vi "Connect Core.vi"(4 "queueRef":refnum<queue>, 5 "Commit Only?":bool, 6 "Access (R/W allowed)":T1, 7 "Mode (buffer)":u16(ring)=1 items=["commit", "buffer"], 8 "Error In":errorcluster, 11 "SVConnection in":refnum<class "DSConnection.lvclass">) -> (0 "Error Out":errorcluster, 3 "SVConnection out":refnum<class "DSConnection.lvclass">)   [LabVIEW 2015, in "CS++ProcessVariables.lvlib" / "DSConnection.lvclass"]
doc: "Open reference to a data socket item if not already connected."
uses:
  DSConnection.lvclass
  DSConnection.lvclass/DSConnection.ctl
  PVConnection/PVConnection.lvclass/PVConnection.ctl
  ProcessVariable/PV.lvclass/PV.ctl
  ProcessVariable/PV.lvclass
  PVConnection/PVConnection.lvclass
  Libraries/Utilities/CS++Utilities.lvlib
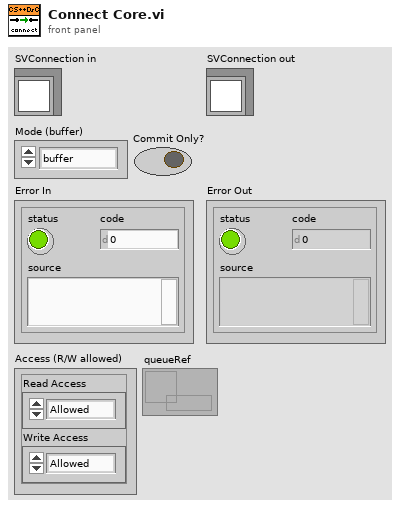
[diagram p1: front panel]
types:
  T1 = cluster{"Read Access":enum8{"Allowed", "Required", "None"}, "Write Access":enum8{"Allowed", "Required", "None"}}
  T2 = enum16{"Read", "Write", "ReadWrite", "BufferedRead", "BufferedReadWrite"}
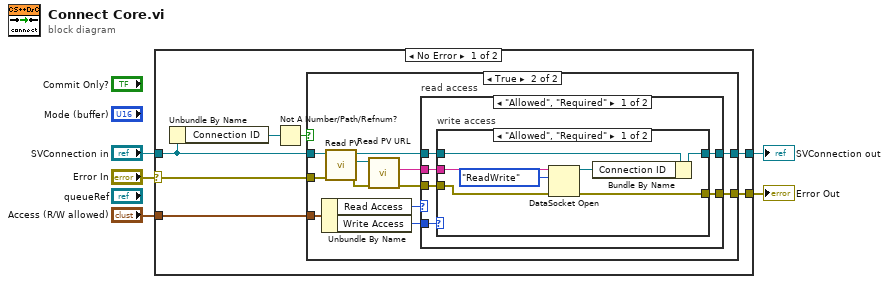
[diagram p0: block diagram]
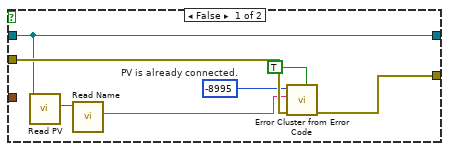
[diagram p2: hidden frame]
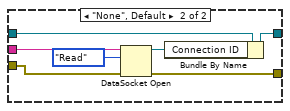
[diagram p3: hidden frame]
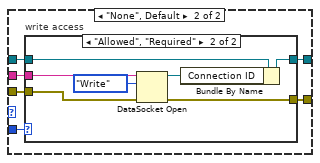
[diagram p4: hidden frame]
diagram:
  n1 = case shown="No Error" "Error In" {
    selector: "Error In" -> [w12 w68]
    tunnel: [w11 w68] -> w4
    tunnel: [w10 w67] -> w2
    tunnel: "SVConnection in" -> [w7 w67]
    tunnel: "Access (R/W allowed)" -> [w8 _]
    frame No Error {
      n2 = Unbundle By Name(w7) -> ("Connection ID"=w6:refnum<k13>)
      n3 = Not A Number/Path/Refnum?(number/path/refnum=w6) -> (NaN/Path/Refnum?=w9:bool)
      n4 = case shown="True" w9 {
        tunnel: w12 -> [w19 w26]
        tunnel: [w18 w31] -> w11
        tunnel: [w15 w30] -> w10
        tunnel: w7 -> [w15 w29]
        tunnel: w8 -> [_ w22]
        frame False {
          w16 = -8995  # PV is already connected.
          n5 = call "Read PV.vi"("PVConnection in"=w15) -> ("PV"=w14:refnum<class "PV.lvclass">)  [unwired: 8 in, 2 out]
          n6 = call "Read Name.vi"("PV in"=w14) -> ("Name"=w13:string)  [unwired: 8 in, 2 out]
          n7 = call "Error Cluster from Error Code.vi"("is warning? (False)"=TRUE ("show call chain? (False)"), "Error In"=w19, "Error Message (\"\")"=w13, "Error Code (0)"=w16) -> ("Error Out"=w18:errorcluster)  [unwired: 7 in]
        }
        frame True {
          n8 = Unbundle By Name(w22) -> ("Read Access"=w21:enum8{"Allowed", "Required", "None"}, "Write Access"=w20:enum8{"Allowed", "Required", "None"})
          n9 = call "Read PV.vi"("error in (no error)"=w26, "PVConnection in"=w29) -> ("error out"=w27:errorcluster, "PV"=w28:refnum<class "PV.lvclass">, "PVConnection out"=w25:refnum<class "DSConnection.lvclass">)  [unwired: 7 in]
          n10 = call "Read PV URL.vi"("error in (no error)"=w27, "PV in"=w28) -> ("error out"=w23:errorcluster, "PV URL"=w24:string)  [unwired: 7 in, 1 out]
          n11 = case "read access" shown="\"Allowed\", \"Required\"" w21 {
            tunnel: [w37 w57] -> w31
            tunnel: [w36 w56] -> w30
            tunnel: w25 -> [w35 w55]
            tunnel: w24 -> [w34 w54]
            tunnel: w23 -> [w33 w53]
            tunnel: w20 -> [w32 w52]
            frame "Allowed", "Required" {
              n12 = case "write access" shown="\"Allowed\", \"Required\"" w32 {
                tunnel: [w44 w51] -> w37
                tunnel: [w43 w50] -> w36
                tunnel: w35 -> [w42 w49]
                tunnel: w34 -> [w41 w48]
                tunnel: w33 -> [w40 w47]
                frame "Allowed", "Required" {
                  n13 = DataSocket Open(8:w40, 10:T2."ReadWrite" ("mode"), 11:w41) -> (0:w44:errorcluster, 3:w39:refnum<k13>)  [unwired: 1 in]
                  n14 = Bundle By Name(cluster=w42, "Connection ID"=w39) -> (w43:refnum<class "DSConnection.lvclass">)
                }
                frame "None", Default {
                  n15 = DataSocket Open(8:w47, 10:T2."Read" ("mode"), 11:w48) -> (0:w51:errorcluster, 3:w46:refnum<k13>)  [unwired: 1 in]
                  n16 = Bundle By Name(cluster=w49, "Connection ID"=w46) -> (w50:refnum<class "DSConnection.lvclass">)
                }
              }
            }
            frame "None", Default {
              n17 = case "write access" shown="\"Allowed\", \"Required\"" w52 {
                tunnel: [w58 w66] -> w57
                tunnel: [w59 w65] -> w56
                tunnel: w55 -> [w59 w64]
                tunnel: w54 -> [_ w63]
                tunnel: w53 -> [w58 w62]
                frame "None", Default {
                }
                frame "Allowed", "Required" {
                  n18 = DataSocket Open(8:w62, 10:T2."Write" ("mode"), 11:w63) -> (0:w66:errorcluster, 3:w61:refnum<k13>)  [unwired: 1 in]
                  n19 = Bundle By Name(cluster=w64, "Connection ID"=w61) -> (w65:refnum<class "DSConnection.lvclass">)
                }
              }
            }
          }
        }
      }
    }
    frame Error {
    }
  }
  "Error Out" <- w4
  "SVConnection out" <- w2
